vi "test Update Discrete Bit Field.vi"(8 "error in (no error)":errorcluster, 11 "TestCase in":refnum<class "Discrete.lvclass">) -> (0 "error out":errorcluster, 3 "TestCase out":refnum<class "Discrete.lvclass">)   [LabVIEW 2020, in "Discrete.lvclass"]
uses:
  Discrete.lvclass
  6e1d2ac8-71cc-41db-b083-493d6063b283.vi
  6e1d2ac8-71cc-41db-b083-493d6063b283.vi/9935dc85-f143-411c-b80b-16b6c96eb14a.vi
  <vilib>/addons/_JKI Toolkits/VI Tester/TestCase.llb/TestCase.lvclass
  C:/Program Files (x86)/National Instruments/LabVIEW 2020/vi.lib/addons/_JKI Toolkits/VI Tester/TestCase.llb/TestCase.lvclass
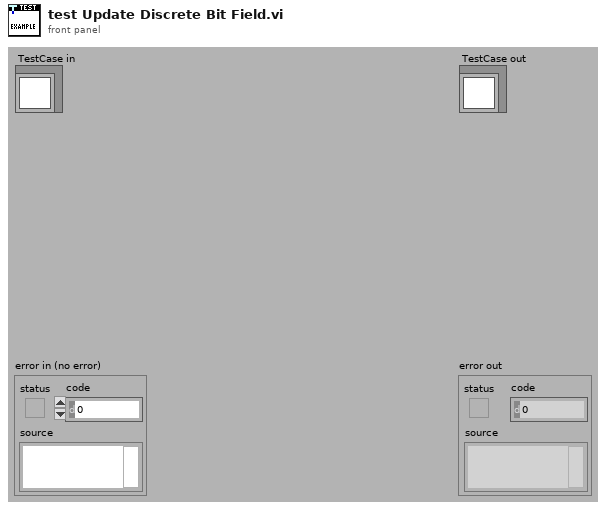
[diagram p1: front panel]
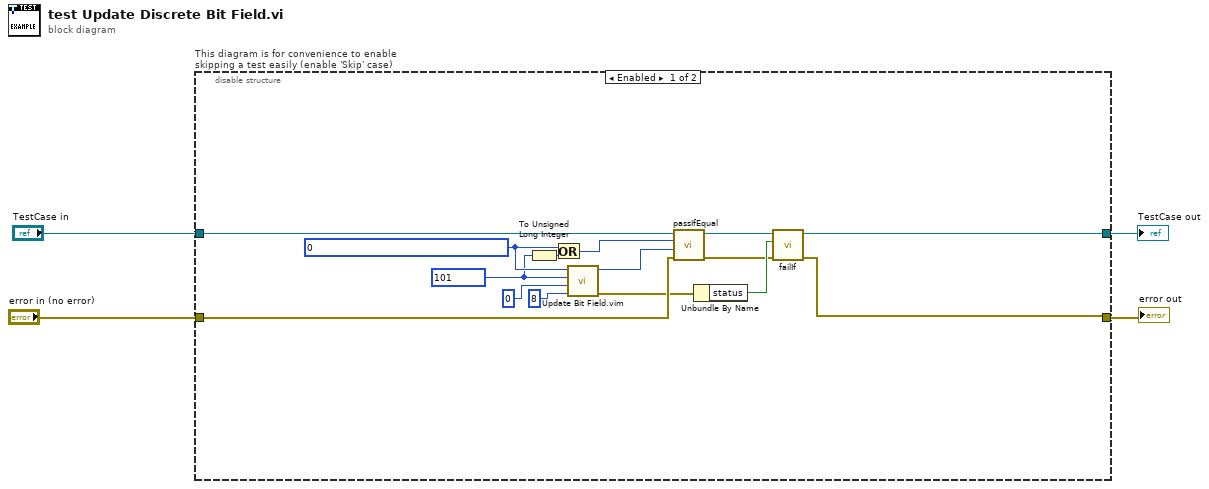
[diagram p0: block diagram]
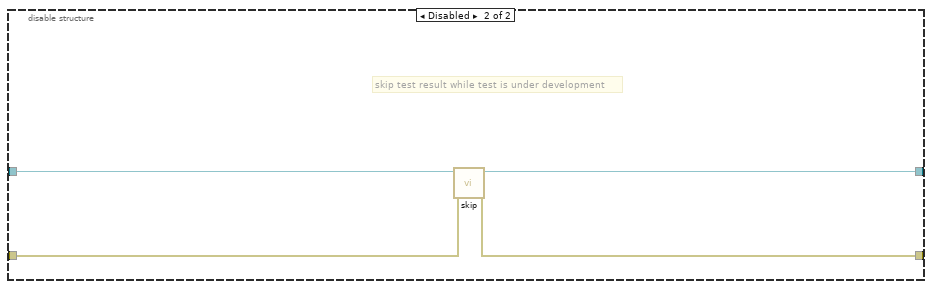
[diagram p2: hidden frame]
diagram:
  n1 = disable-structure "This diagram is for convenience to enable skipping a test easily (enable 'Skip' case)" shown="Enabled" {
    disable-tunnel: "TestCase in" -> [w19 w23]
    disable-tunnel: [w5 w21] -> w1
    disable-tunnel: [w6 w22] -> w3
    disable-tunnel: "error in (no error)" -> [w11 w20]
    frame Enabled {
      w15 = u8 101 ("value")
      w16 = u32 0 ("word in")
      n2 = To Unsigned Long Integer(number=w15) -> (unsigned 32bit integer=w14:u32)
      n3 = Or(x=w16, y=w14) -> (x .or. y?=w13:u32)
      n4 = call "Update Bit Field.vim"("bit field size"=8, "bit field start index"=0, "value"=w15, "word in"=w16) -> ("error out"=w10:errorcluster, "word out"=w12:u32)  [unwired: 6 in]
      n5 = call-dynamic "passIfEqual.vi"("error in (no error)"=w11, "y"=w12, "x"=w13, "TestCase in"=w19) -> ("error out"=w7:errorcluster, "TestCase out"=w8:refnum<class "Discrete.lvclass">)  [unwired: 6 in]
      n6 = Unbundle By Name(w10) -> ("status"=w9:bool)
      n7 = call-dynamic "failIf.vi"("error in (no error)"=w7, "fail"=w9, "TestCase in"=w8) -> ("error out"=w6:errorcluster, "TestCase out"=w5:refnum<class "Discrete.lvclass">)  [unwired: 7 in]
    }
    frame Disabled {
      # "skip test result while test is under development"
      n8 = call <vilib>:"skip.vi"("error in (no error)"=w20, "TestCase in"=w23) -> ("error out"=w22:errorcluster, "TestCase out"=w21:refnum<class "Discrete.lvclass">)  [unwired: 8 in]
    }
  }
  "error out" <- w3
  "TestCase out" <- w1
